vi "Error Message Manager.vi"(8 "error in":errorcluster, 9 "Variable Msg":string[](array[string]), 11 "Error Selection":T1=enum."Duplicated GU Number") -> (0 "error out":errorcluster)   [LabVIEW 2020, in "GUCalibration2.lvlib"]
uses:
  GUCalibration2.lvlib
  Controls/Error Enum.ctl
  <vilib>/Utility/error.llb/DialogType.ctl
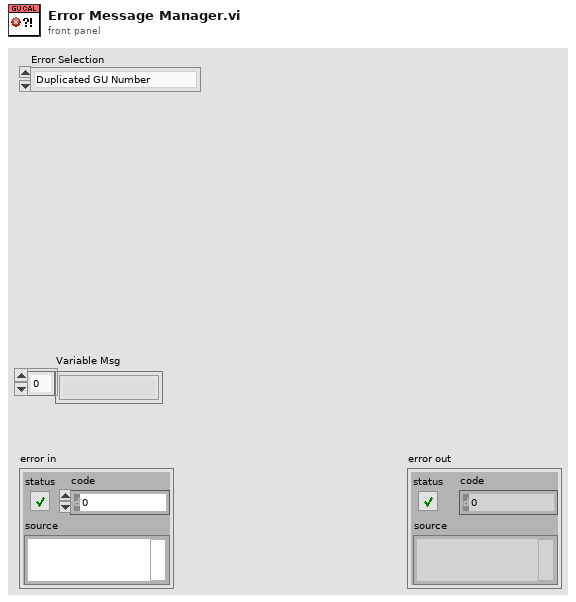
[diagram p1: front panel]
types:
  T1 = typedef "GUCalibration2.lvlib/Error Enum.ctl" = enum16{"Error Template Case", "Duplicated GU Number", "Test Items Mismatch"}
  T2 = typedef "DialogType.ctl" = u16
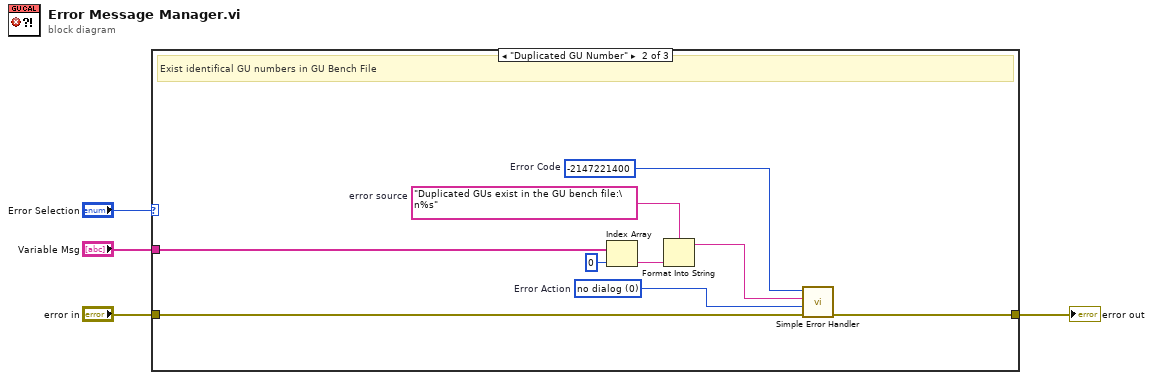
[diagram p0: block diagram]
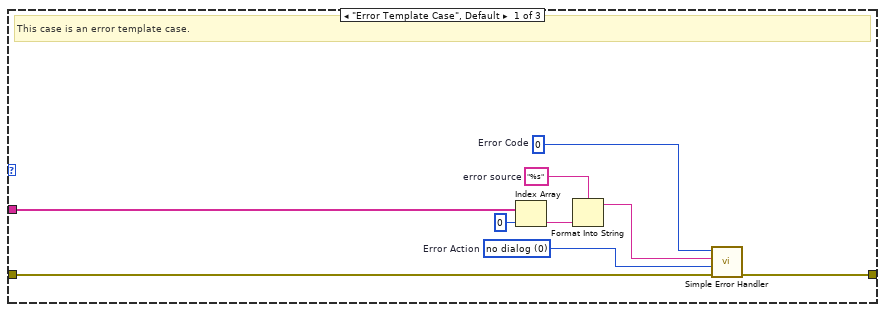
[diagram p2: hidden frame]
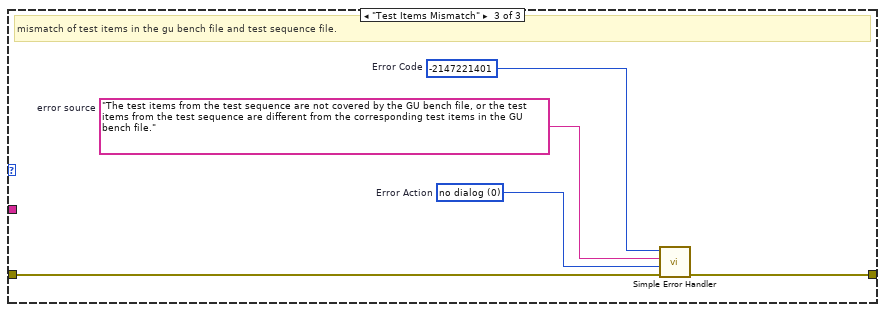
[diagram p3: hidden frame]
diagram:
  n1 = case shown="\"Duplicated GU Number\"" "Error Selection" {
    tunnel: [w10 w19 w24] -> w3
    tunnel: "error in" -> [w11 w20 w25]
    tunnel: "Variable Msg" -> [w8 w17 _]
    frame "Error Template Case", Default {
      w9 = "%s"  # error source
      w12 = 0  # Error Code
      w13 = T2 0 items=["no dialog", "OK message", "continue or stop message", "OK message + warnings", "continue/stop + warnings"]  # Error Action
      # "This case is an error template case."
      n2 = Index Array(array=w8, index=0) -> (element=w6:string)
      n3 = Format Into String(format string=w9, w6) -> (resulting string=w5:string)  [unwired: 2 in, 1 out]
      n4 = call <vilib>:"Simple Error Handler.vi"("error code (no error:0)"=w12, "error source (\" \")"=w5, "type of dialog (OK msg:1)"=w13, "error in (no error)"=w11) -> ("error out"=w10:errorcluster)  [unwired: 1 in, 4 out]
    }
    frame "Duplicated GU Number" {
      w18 = "Duplicated GUs exist in the GU bench file:\n%s"  # error source
      w21 = -2147221400  # Error Code
      w22 = T2 0 items=["no dialog", "OK message", "continue or stop message", "OK message + warnings", "continue/stop + warnings"]  # Error Action
      # "Exist identifical GU numbers in GU Bench File"
      n5 = Index Array(array=w17, index=0) -> (element=w15:string)
      n6 = Format Into String(format string=w18, w15) -> (resulting string=w14:string)  [unwired: 2 in, 1 out]
      n7 = call <vilib>:"Simple Error Handler.vi"("error code (no error:0)"=w21, "error source (\" \")"=w14, "type of dialog (OK msg:1)"=w22, "error in (no error)"=w20) -> ("error out"=w19:errorcluster)  [unwired: 1 in, 4 out]
    }
    frame "Test Items Mismatch" {
      w23 = "The test items from the test sequence are not covered by the GU bench file, or the test items from the test sequence are different from the corresponding test items in the GU bench file."  # error source
      w26 = -2147221401  # Error Code
      w27 = T2 0 items=["no dialog", "OK message", "continue or stop message", "OK message + warnings", "continue/stop + warnings"]  # Error Action
      # "mismatch of test items in the gu bench file and test sequence file."
      n8 = call <vilib>:"Simple Error Handler.vi"("error code (no error:0)"=w26, "error source (\" \")"=w23, "type of dialog (OK msg:1)"=w27, "error in (no error)"=w25) -> ("error out"=w24:errorcluster)  [unwired: 1 in, 4 out]
    }
  }
  "error out" <- w3
